vi "Abort.vi"(8 "error in (no error)":errorcluster, 11 "PacificPowerSource in":refnum<class "PacificPowerSource.lvclass">) -> (0 "error out":errorcluster, 3 "PacificPowerSource out":refnum<class "PacificPowerSource.lvclass">)   [LabVIEW 2018, in "AcPwrPlugins.lvlib" / "PacificPowerSource.lvclass"]
uses:
  PacificPowerSource.lvclass
  AcPwrBaseClass/AcPwrBase.lvclass
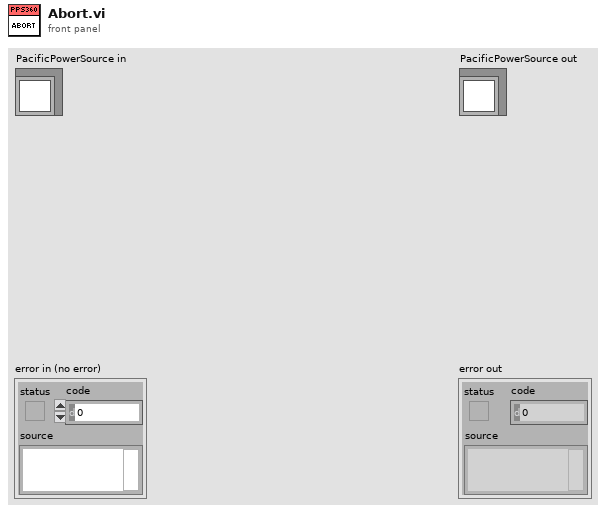
[diagram p1: front panel]
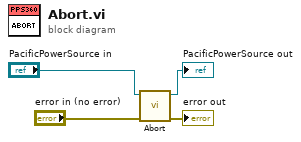
[diagram p0: block diagram]
diagram:
  n1 = call-parent "Abort.vi"("error in (no error)"="error in (no error)", "AcPwrBase in"="PacificPowerSource in") -> ("error out"=→"error out":errorcluster, "AcPwrBase out"=→"PacificPowerSource out":refnum<class "PacificPowerSource.lvclass">)  [unwired: 8 in]
